vi "Pulse Control.vi"() -> ()   [LabVIEW 2012]
panel:
  in  "Stop Button":bool
  out "Output":dbl(graph)
  in  "BPM":dbl(slide)=60.0 min=0.0 max=200.0 step=5.0 scale=0.0..200.0
  in  "Min Voltage":dbl(slide)=6.0 min=0.0 max=18.0 step=0.5 scale=0.0..18.0
  in  "Max Voltage":dbl(slide)=12.0 min=0.0 max=18.0 step=0.5 scale=0.0..18.0
  in  "Duty Cycle":dbl(slide)=0.30000000000000004 min=0.0 max=1.0 step=0.1 scale=0.0..1.0
  in  "Loop Delay (ms)":u32=50
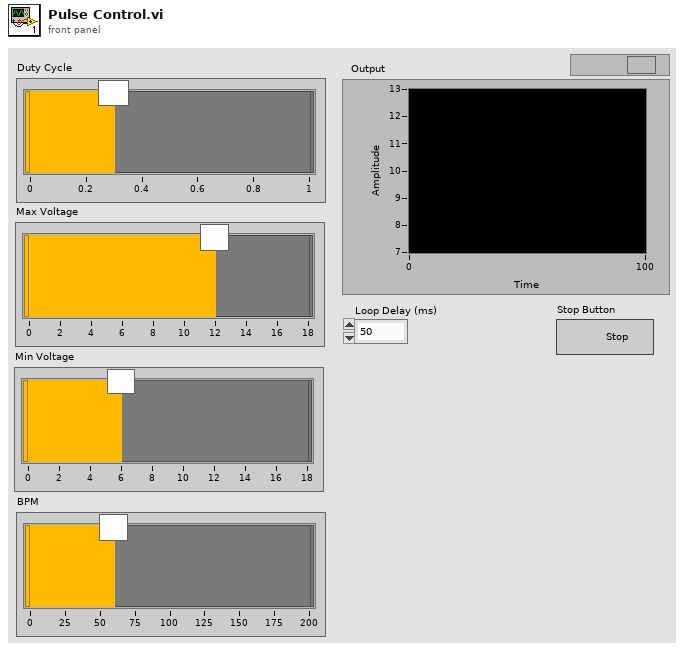
[diagram p1: front panel]
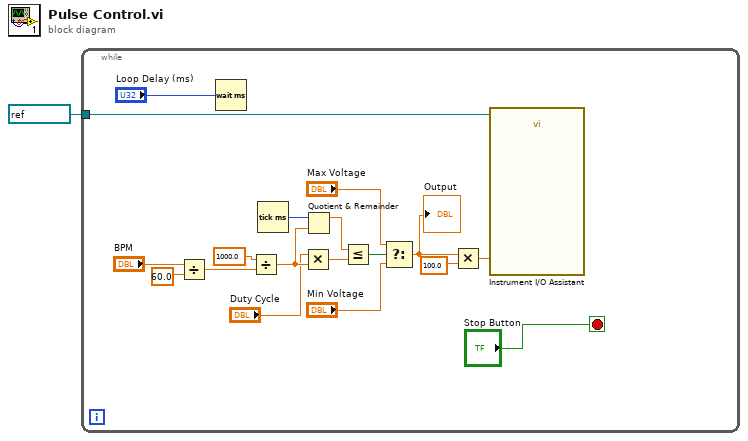
[diagram p0: block diagram]
diagram:
  n1 = while {
    tunnel: refnum<visa-resource-name> "COM5" ("Session In") -> [w18]
    stop <- "Stop Button" stop-if-true
    n2 = Divide(x="BPM", y=60.0) -> (x/y=w13:dbl)
    n3 = Wait (ms)(milliseconds to wait="Loop Delay (ms)") -> ()  [unwired: 1 out]
    n4 = Divide(x=1000.0, y=w13) -> (x/y=w11:dbl)
    n5 = Tick Count (ms)() -> (millisecond timer value=w12:u32)
    n6 = Multiply(x="Duty Cycle", y=w11) -> (x*y=w9:dbl)
    n7 = Quotient & Remainder(x=w12, y=w11) -> (x-y*floor(x/y)=w10:dbl)  [unwired: 1 out]
    n8 = Less Or Equal?(x=w10, y=w9) -> (x <= y?=w8:bool)
    n9 = Select(t="Max Voltage", s=w8, f="Min Voltage") -> (s? t:f=w5:dbl)
    "Output" <- w5
    n10 = Multiply(x=w5, y=100.0) -> (x*y=w15:dbl)
    n11 = call "Instrument I/O Assistant"("Session In"=w18, "voltage"=w15) -> ()  [unwired: 24 in, 2 out]
  }
